vi "HEAD.vi"(6 "timeout":i32=10000, 8 "error in":errorcluster, 10 "url":string, 11 "http-method in":refnum<class "REST Client.lvclass">) -> (0 "error out":errorcluster, 2 "response":refnum<class "response.lvclass">, 3 "http-method out":refnum<class "REST Client.lvclass">)   [LabVIEW 2020, in "REST Client.lvlib" / "REST Client.lvclass"]
uses:
  REST Client.lvclass
  response/response.lvclass
  http-client/http-client.lvclass
  REST Client.lvclass/REST Client.ctl
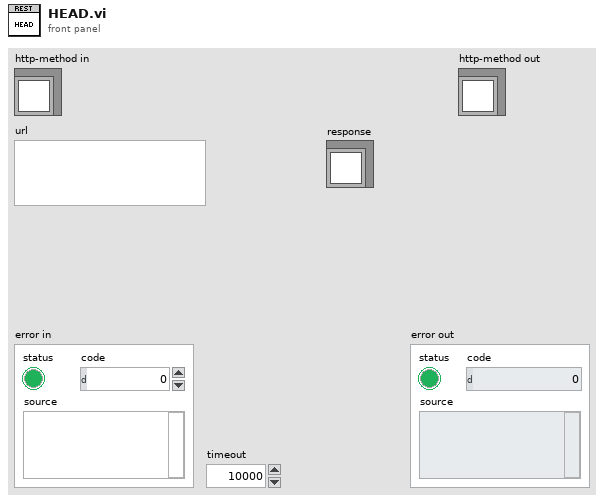
[diagram p1: front panel]
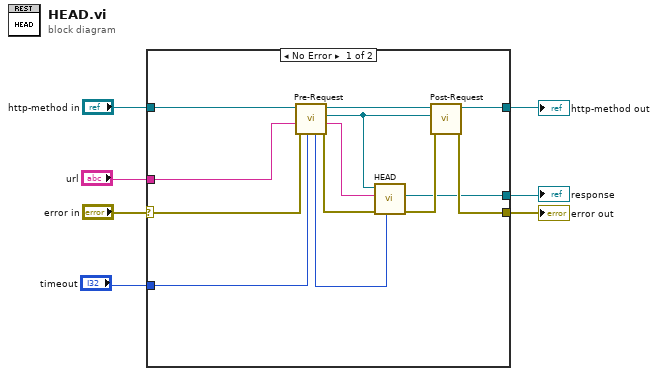
[diagram p0: block diagram]
diagram:
  n1 = case shown="No Error" "error in" {
    selector: "error in" -> [w16 w22]
    tunnel: [w13 w22] -> w1
    tunnel: [w14 w21] -> w2
    tunnel: "http-method in" -> [w15 w21]
    tunnel: "url" -> [w10 _]
    tunnel: "timeout" -> [w9 _]
    tunnel: [w12 _] -> w3
    frame No Error {
      n2 = call "Pre-Request.vi"("timeout"=w9, "error in (no error)"=w16, "url"=w10, "REST Client in"=w15) -> ("error out"=w18:errorcluster, "Resolved URL"=w11:string, "http-client"=w19:refnum<class "http-client.lvclass">, "REST Client out"=w20:refnum<class "REST Client.lvclass">, "Timeout"=w8:i32)  [unwired: 3 in]
      n3 = call-dynamic "HEAD.vi"("timeout"=w8, "error in"=w18, "url"=w11, "http-method in"=w19) -> ("error out"=w17:errorcluster, "response"=w12:refnum<class "response.lvclass">)  [unwired: 5 in, 1 out]
      n4 = call "Post-Request.vi"("error in (no error)"=w17, "http-method in"=w19, "REST Client in"=w20) -> ("error out"=w13:errorcluster, "REST Client out"=w14:refnum<class "REST Client.lvclass">)  [unwired: 7 in]
    }
    frame Error {
    }
  }
  "error out" <- w1
  "http-method out" <- w2
  "response" <- w3
